vi "SeCrTs-CS Log Digital Queues.vi"(8 "error in":errorcluster, 9 "DI_queue":refnum<queue>[](array[refnum]), 10 "DI Names":string[](array[string]), 11 "tdms file in":refnum<k34>) -> (0 "error out":errorcluster, 3 "tdms file out":refnum<k34>)   [LabVIEW 2022 SP3]
uses:
  <vilib>/Waveform/DWDTOps.llb/DWDT Digital to Analog.vi
  <vilib>/Waveform/DWDTOps.llb/DWDT Get Waveform Time Array.vi
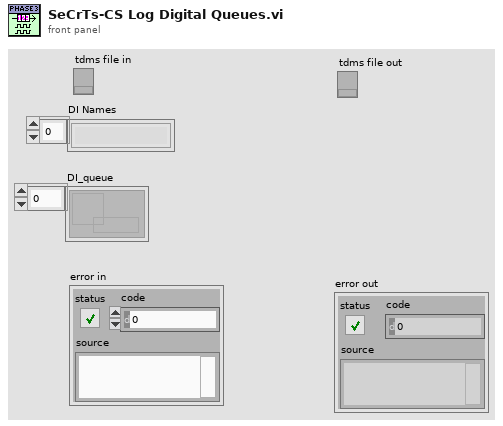
[diagram p1: front panel]
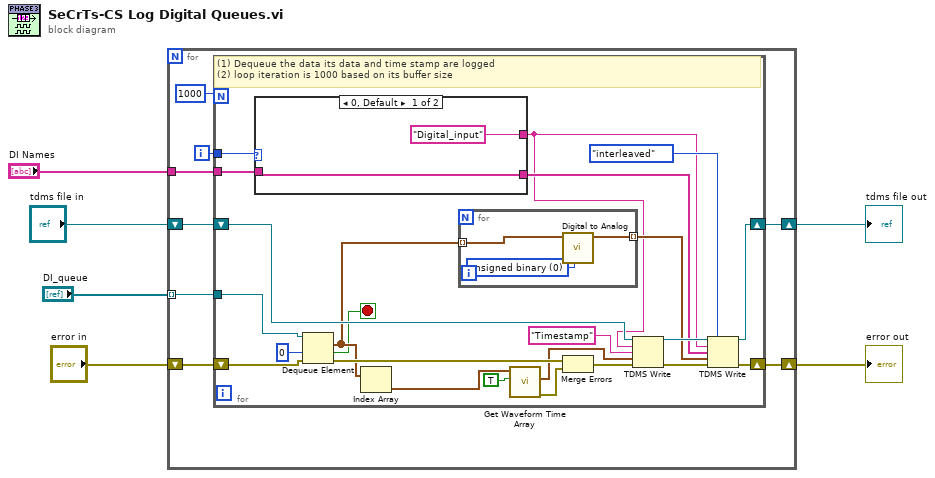
[diagram p0: block diagram]
diagram:
  n1 = for {
    tunnel: "DI_queue" -> [w11] mode=indexing
    tunnel: "DI Names" -> [w8]
    shift-right: [w9] -> w2
    shift-left: "error in" -> [w14]
    shift-right: [w10] -> w3
    shift-left: "tdms file in" -> [w13]
    i -> [w7]
    n2 = for {
      N: 1000 -> [_]
      shift-right: [w26] -> w10
      shift-left: w13 -> [w28]
      shift-right: [w31] -> w9
      shift-left: w14 -> [w34]
      tunnel: w11 -> [w19]
      tunnel: w8 -> [w18]
      tunnel: w7 -> [w17]
      stop <- w22 stop-if-true
      # "(1) Dequeue the data its data and time stamp are logged\n(2) loop iteration is 1000 based on its buffer size"
      n3 = case shown="0, Default" w17 {
        tunnel: w18 -> [w39 _]
        tunnel: [w39 _] -> w16
        tunnel: ["Digital_input" ("group name in (Untitled)") _] -> w15
        frame 0, Default {
        }
        frame 1 {
        }
      }
      n4 = Dequeue Element(queue=w19, timeout in ms (-1)=0, error in (no error)=w34) -> (element=w24:digitalwaveform[], timed out?=w22:bool, error out=w36:errorcluster)  [unwired: 1 out]
      n5 = Index Array(array=w24) -> (element=w20:digitalwaveform)  [unwired: 1 in]
      n6 = for {
        tunnel: w24 -> [w42] mode=indexing
        tunnel: [w41] -> w23 mode=indexing
        w40 = u16 0 items=["unsigned binary", "offset binary", "2's complement"] ("data format (offset binary)")
        n7 = call-poly <vilib>:"Digital to Analog.vi"("data format (offset binary)"=w40, "digital waveform"=w42) -> ("analog waveform"=w41:waveform(dbl))  [unwired: 6 in, 3 out]
      }
      n8 = call-poly <vilib>:"Get Waveform Time Array.vi"("match transition array"=TRUE, "waveform in"=w20) -> ("error out"=w35:errorcluster, "X array"=w29:timestamp[])  [unwired: 8 in]
      n9 = Merge Errors(w36, w35) -> (w33:errorcluster)
      n10 = TDMS Write(0:w28, 5:w15, 7:"Timestamp", 9:w29, 11:w33) -> (4:w27:refnum<k34>, 15:w32:errorcluster)  [unwired: 1 in, 2 out]
      n11 = TDMS Write(0:w27, 1:enum16{"decimated", "interleaved"}."interleaved" ("data layout (0:decimated)"), 5:w15, 7:w16, 9:w23, 11:w32) -> (4:w26:refnum<k34>, 15:w31:errorcluster)  [unwired: 2 out]
    }
  }
  "tdms file out" <- w3
  "error out" <- w2
